vi "Terminate.vi"(6 "Teller":refnum<class "Teller.lvclass">, 9 "Error":errorcluster, 10 "Actor":refnum<class "Actor.lvclass">, 11 "Core Actor in":refnum<class "Core Actor.lvclass">) -> (0 "Error out":errorcluster, 3 "Core Actor out":refnum<class "Core Actor.lvclass">)   [LabVIEW 2025, in "jettl.lvlib" / "Actor.lvlib" / "Core Actor.lvclass"]
uses:
  Core Actor.lvclass
  C:/git/jettl/src/jettl/jettl/Actor/Actor/Actor.lvclass
  Actor/Actor.lvclass
  Teller/Teller/Teller.lvclass
  Core Actor.lvclass/Core Actor.ctl
  Stop Msg/Direct Call.vi
  Attributes/Attributes/Attributes.lvclass
  Stop Msg/Stop Msg.lvlib
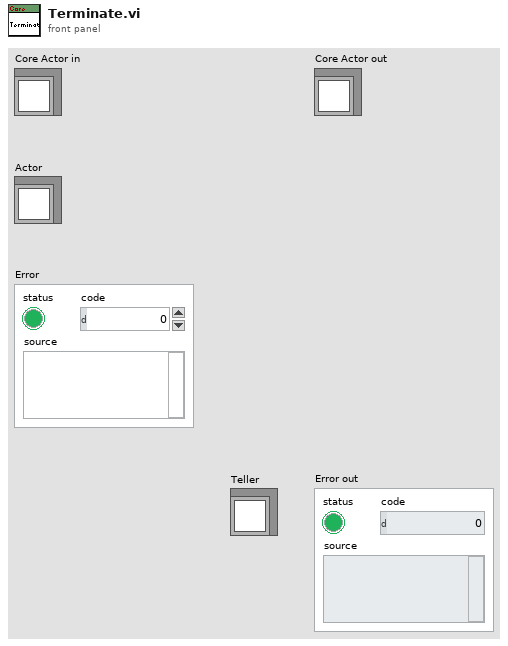
[diagram p1: front panel]
types:
  T1 = typedef "jettl.lvlib/Actor.lvlib/Relation.ctl" = enum16{"Self", "Parent", "Child"}
  T2 = typedef "jettl.lvlib/Actor.lvlib/Core Actor.lvclass/Child Attributes Map.ctl" = map{string, refnum<class "Attributes.lvclass">}
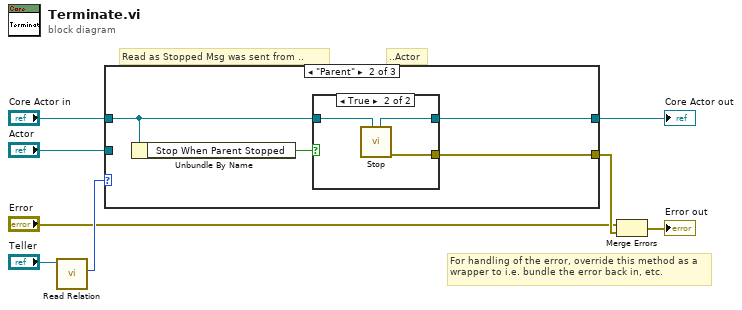
[diagram p0: block diagram]
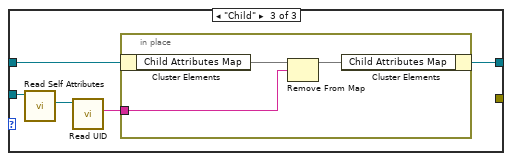
[diagram p4: hidden frame]
diagram:
  # "For handling of the error, override this method as a wrapper to i.e. bundle the error back in, etc."
  # "..Actor"
  # "Read as Stopped Msg was sent from .."
  n1 = call-dynamic "Read Relation.vi"("Teller in"="Teller") -> ("Relation"=w4:T1)  [unwired: 10 in]
  n2 = case shown="\"Parent\"" w4 {
    tunnel: "Core Actor in" -> [w9 w11 w21]
    tunnel: [w9 w13 w18] -> w8
    tunnel: "Actor" -> [_ _ w22]
    tunnel: [_ w12 _] -> w2
    frame "Self" {
      # "Case will not fundamentally execute"
    }
    frame "Parent" {
      n3 = Unbundle By Name(w11) -> ("Stop When Parent Stopped"=w10:bool)
      n4 = case shown="True" w10 {
        tunnel: [w14 w17] -> w13
        tunnel: [_ w16] -> w12
        tunnel: w11 -> [w14 w15]
        frame False {
        }
        frame True {
          n5 = call-poly "Stop.vi"("Actor in"=w15) -> ("Error out"=w16:errorcluster, "Actor out"=w17:refnum<class "Core Actor.lvclass">)  [unwired: 9 in]
        }
      }
    }
    frame "Child" {
      n6 = call-dynamic "Read Self Attributes.vi"("Actor in"=w22) -> ("Self Attributes"=w20:refnum<class "Attributes.lvclass">)  [unwired: 10 in]
      n7 = call-dynamic "Read UID.vi"("Attributes in"=w20) -> ("UID"=w19:string)  [unwired: 10 in]
      n8 = in-place {
        in-place-border: w19 -> [w23]
        n9 = in-place-cluster #1(w21) -> ("Child Attributes Map"=w25:T2)
        n10 = Remove From Map(10:w23, 11:w25) -> (3:w24:T2)  [unwired: 2 out]
        n11 = in-place-cluster #1("Child Attributes Map"=w24) -> (w18:refnum<class "Core Actor.lvclass">)
      }
    }
  }
  "Core Actor out" <- w8
  n12 = Merge Errors("Error", w2) -> (→"Error out":errorcluster)
